vi "Demo - Test Message Sequence.vi"() -> ()   [LabVIEW 2020]
panel:
  out "Received Message Array":string[](array[string])
  in  "Port":u16=9760
  in  "IP Address - DAQ":string="192.168.1.1"
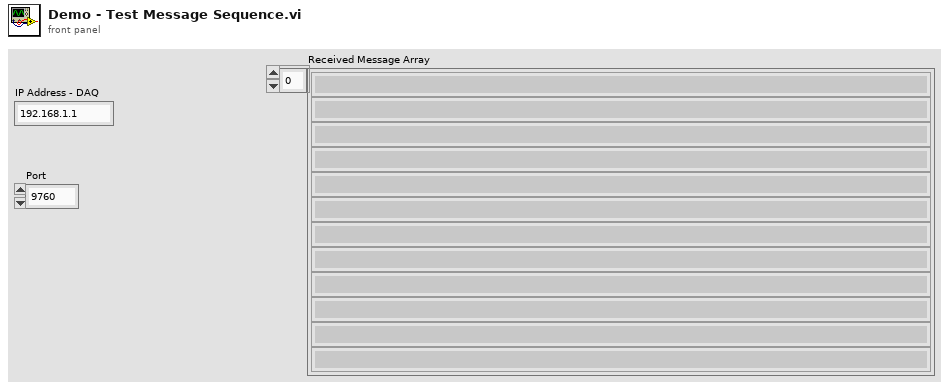
[diagram p1: front panel]
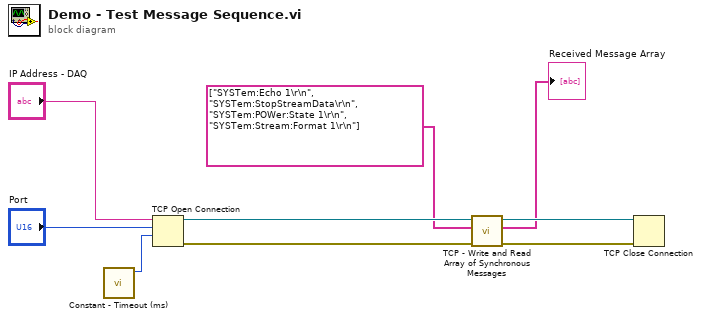
[diagram p0: block diagram]
diagram:
  n1 = call "Constant - Timeout (ms).vi"() -> ("timeout (ms)"=w5:i32)  [unwired: 11 in]
  n2 = TCP Open Connection(address="IP Address - DAQ", remote port or service name="Port", timeout ms (60000)=w5) -> (connection ID=w7:refnum<k5>, error out=w6:errorcluster)  [unwired: 2 in]
  n3 = call "TCP - Write and Read Array of Synchronous Messages.vi"("error in"=w6, "Array of Messages to Send"=string[] ["SYSTem:Echo 1\r\n", "SYSTem:StopStreamData\r\n", "SYSTem:POWer:State 1\r\n", "SYSTem:Stream:Format 1\r\n"], "TCP Network Connection in"=w7) -> ("error out"=w2:errorcluster, "Received Message Array"=→"Received Message Array":string[], "TCP Network Connection out"=w3:refnum<k5>)  [unwired: 6 in]
  n4 = TCP Close Connection(connection ID=w3, error in (no error)=w2) -> ()  [unwired: 1 in, 2 out]
